vi "Flatness Out of The Box.vi"() -> ()   [LabVIEW 2017]
uses:
  <vilib>/Analysis/1siggen.llb/Ramp Pattern by Delta.vi
  <vilib>/Analysis/NI_AALBase.lvlib
panel:
  out "XY Graph 3":cluster{dbl[], dbl[]}(graph)
  out "XY Graph 2":cluster{dbl[], dbl[]}(graph)
  out "XY Graph":cluster{dbl[], dbl[]}(graph)
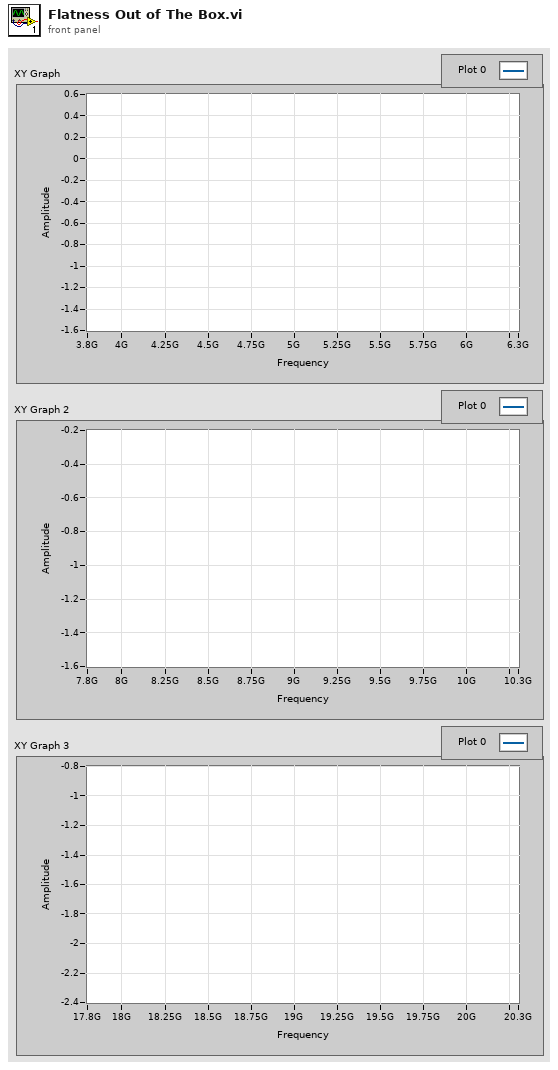
[diagram p1: front panel]
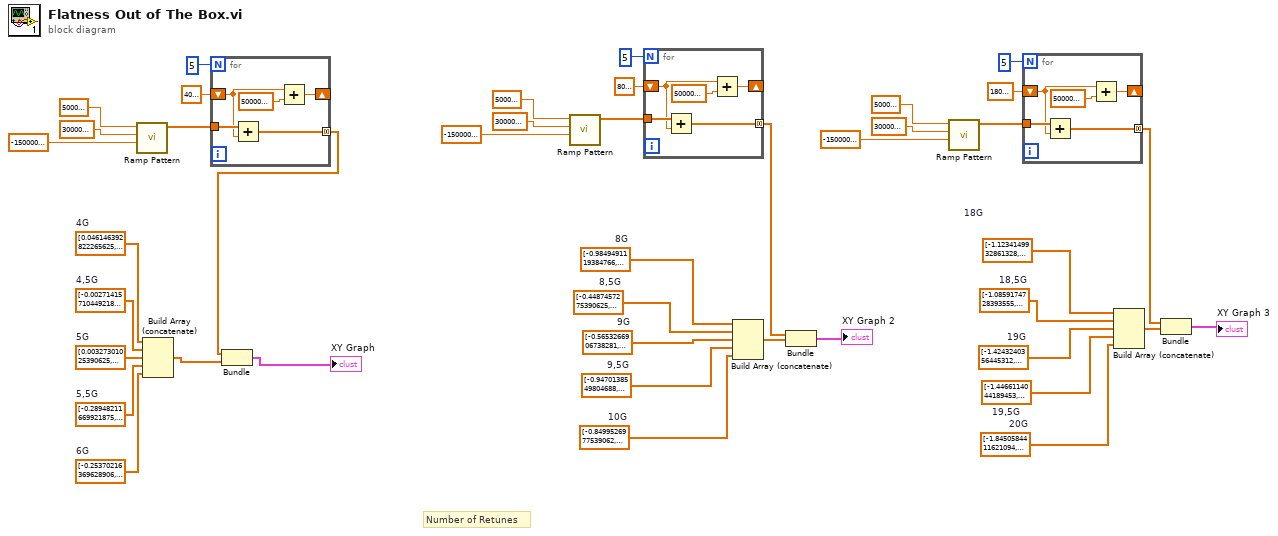
[diagram p0: block diagram]
diagram:
  w10 = dbl[] [-1.8450584411621094, -2.2662086486816406, -2.00801944732666, -1.8645620346069336, -1.6340160369873047, -1.6154193878173828, -1.5437860488891602, -1.7546768188476562, -1.8310136795043945, -1.5069427490234375]  # 20G
  w11 = dbl[] [-1.4466114044189453, -1.7337331771850586, -1.6114177703857422, -1.6368112564086914, -1.404719352722168, -1.4472150802612305, -1.6012763977050781, -1.9720754623413086, -1.9070043563842773, -1.6358604431152344]  # 19,5G
  w12 = dbl[] [-1.4243240356445312, -1.6523551940917969, -1.6257820129394531, -1.586716651916504, -1.3976774215698242, -1.5765323638916016, -1.6395072937011719, -1.8030452728271484, -2.0713062286376953, -1.5772209167480469]  # 19G
  w13 = dbl[] [-1.0859174728393555, -1.445211410522461, -1.3843650817871094, -1.2820110321044922, -1.115631103515625, -1.2875919342041016, -1.3207368850708008, -1.6865196228027344, -1.7107582092285156, -1.444925308227539]  # 18,5G
  w14 = dbl[] [-1.1234149932861328, -1.4323577880859375, -1.3264636993408203, -1.5126972198486328, -1.2935047149658203, -1.2274208068847656, -1.4697589874267578, -1.5328483581542969, -1.4974756240844727, -0.8757257461547852]  # 18G
  w24 = dbl[] [-0.8499526977539062, -1.005141258239746, -1.2255582809448242, -1.3272132873535156, -1.1354122161865234, -1.0941829681396484, -1.2211322784423828, -1.5586128234863281, -1.4991865158081055, -1.1140518188476562]  # 10G
  w25 = dbl[] [-0.9470138549804688, -1.4711933135986328, -1.0435762405395508, -0.9760198593139648, -1.0578670501708984, -1.2179803848266602, -1.0357494354248047, -0.9843606948852539, -1.1925535202026367, -0.9204683303833008]  # 9,5G
  w26 = dbl[] [-0.5653266906738281, -1.0669994354248047, -1.1604557037353516, -1.1625299453735352, -0.700164794921875, -0.7524738311767578, -0.992579460144043, -1.151437759399414, -0.9839324951171875, -0.3832740783691406]  # 9G
  w27 = dbl[] [-0.4487457275390625, -0.6148519515991211, -0.8186206817626953, -0.8637371063232422, -0.5958995819091797, -0.5837583541870117, -0.9039249420166016, -1.3068675994873047, -1.2749252319335938, -0.7583351135253906]  # 8,5G
  w28 = dbl[] [-0.9849491119384766, -0.9787502288818359, -0.6777915954589844, -0.9394187927246094, -0.7365303039550781, -0.7333364486694336, -0.7470817565917969, -1.050210952758789, -1.263214111328125, -0.7880420684814453]  # 8G
  w39 = dbl[] [-0.28948211669921875, -0.7322025299072266, -0.34381866455078125, -0.11953544616699219, -0.4343719482421875, -0.7089214324951172, -0.6704854965209961, -0.6076164245605469, -0.9670591354370117, -1.1165046691894531]  # 5,5G
  w38 = dbl[] [-0.25370216369628906, -0.1826801300048828, -0.2269916534423828, -0.5991401672363281, -0.6511831283569336, -0.5334053039550781, -0.5634002685546875, -1.1348533630371094, -1.3019466400146484, -0.5775814056396484]  # 6G
  w40 = dbl[] [0.00327301025390625, -0.30593299865722656, -0.36382102966308594, -0.4134178161621094, -0.050993919372558594, -0.3513193130493164, -0.6875648498535156, -0.8681859970092773, -0.5846309661865234, -0.1547069549560547]  # 5G
  w41 = dbl[] [-0.0027141571044921875, 0.48984718322753906, 1.1444091796875e-05, -0.2603187561035156, -0.22892475128173828, -0.32309532165527344, -0.4349374771118164, -0.8023691177368164, -0.9535350799560547, -0.4886350631713867]  # 4,5G
  w42 = dbl[] [0.046146392822265625, -0.4790067672729492, -0.4296913146972656, -0.45362186431884766, -0.5820188522338867, -0.9245090484619141, -1.0547065734863281, -1.3147878646850586, -1.4216413497924805, -1.3959617614746094]  # 4G
  # "Number of Retunes"
  n1 = call-poly <vilib>:"Ramp Pattern.vi"("start"=-150000000.0, "end"=300000000.0, "delta"=50000000.0) -> ("Ramp Pattern"=w34:dbl[])  [unwired: 6 in, 2 out]
  n2 = Build Array (concatenate)(w42, w41, w40, w39, w38) -> (w31:dbl[])
  n3 = for {
    N: 5 -> [_]
    tunnel: w34 -> [w47]
    shift-right: [w44] -> _
    shift-left: 4000000000.0 -> [w46]
    tunnel: [w43] -> w30 mode=concatenating
    n4 = Add(x=w47, y=w46) -> (x+y=w43:dbl[])
    n5 = Add(x=w46, y=500000000.0) -> (x+y=w44:dbl)
  }
  n6 = Bundle(w30, w31) -> (→"XY Graph":cluster{dbl[], dbl[]})  [unwired: 1 in]
  n7 = call-poly <vilib>:"Ramp Pattern.vi"("start"=-150000000.0, "end"=300000000.0, "delta"=50000000.0) -> ("Ramp Pattern"=w19:dbl[])  [unwired: 6 in, 2 out]
  n8 = for {
    N: 5 -> [_]
    tunnel: w19 -> [w52]
    shift-right: [w49] -> _
    shift-left: 8000000000.0 -> [w51]
    tunnel: [w48] -> w16 mode=concatenating
    n9 = Add(x=w52, y=w51) -> (x+y=w48:dbl[])
    n10 = Add(x=w51, y=500000000.0) -> (x+y=w49:dbl)
  }
  n11 = Build Array (concatenate)(w28, w27, w26, w25, w24) -> (w23:dbl[])
  n12 = Bundle(w16, w23) -> (→"XY Graph 2":cluster{dbl[], dbl[]})  [unwired: 1 in]
  n13 = call-poly <vilib>:"Ramp Pattern.vi"("start"=-150000000.0, "end"=300000000.0, "delta"=50000000.0) -> ("Ramp Pattern"=w6:dbl[])  [unwired: 6 in, 2 out]
  n14 = for {
    N: 5 -> [_]
    tunnel: w6 -> [w57]
    shift-right: [w54] -> _
    shift-left: 18000000000.0 -> [w56]
    tunnel: [w53] -> w2 mode=concatenating
    n15 = Add(x=w57, y=w56) -> (x+y=w53:dbl[])
    n16 = Add(x=w56, y=500000000.0) -> (x+y=w54:dbl)
  }
  n17 = Build Array (concatenate)(w14, w13, w12, w11, w10) -> (w9:dbl[])
  n18 = Bundle(w2, w9) -> (→"XY Graph 3":cluster{dbl[], dbl[]})  [unwired: 1 in]
